vi "Data Aquired.vi"(8 "error in (no error)":errorcluster, 10 "Data":dbl[](array[numeric]), 11 "Businness Logic in":refnum<class "Businness Logic.lvclass">) -> (0 "error out":errorcluster, 3 "Businness Logic out":refnum<class "Businness Logic.lvclass">)   [LabVIEW 2020, in "Businness Logic.lvlib" / "Businness Logic.lvclass"]
uses:
  Businness Logic.lvclass
  Businness Logic.lvclass/Businness Logic.ctl
  User Interface Messages/Update Data Msg/Update Data Msg.lvclass
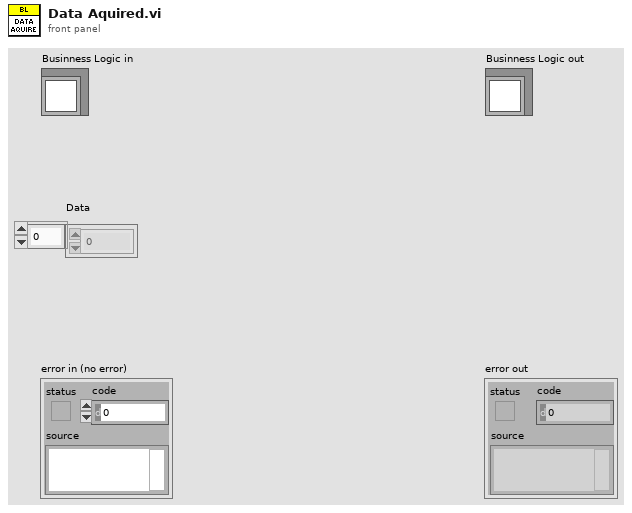
[diagram p1: front panel]
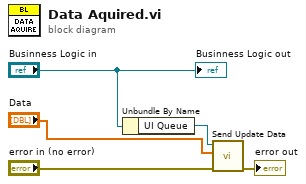
[diagram p0: block diagram]
diagram:
  n1 = Unbundle By Name("Businness Logic in") -> ("UI Queue"=w3:refnum<class "Message Enqueuer.lvclass">)
  n2 = call "Send Update Data.vi"("error in (no error)"="error in (no error)", "Data"="Data", "Message Enqueuer"=w3) -> ("error out"=→"error out":errorcluster)  [unwired: 7 in, 1 out]
  "Businness Logic out" <- "Businness Logic in"
